vi "SV Limit Test (array) (DBL) (No State).vi"(9 "lower limit":dbl, 10 "upper limit":dbl, 11 "Y":dbl[](array[numeric])) -> (1 "lower":T1, 2 "upper":T2, 3 "test passed":bool)   [LabVIEW 2017]
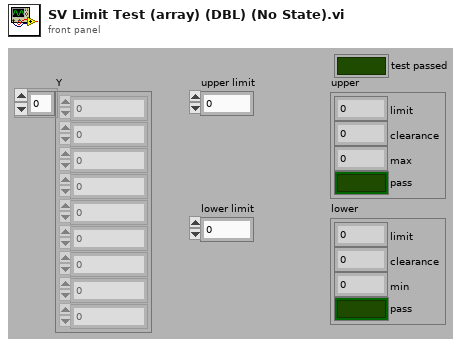
[diagram p1: front panel]
types:
  T1 = cluster{"limit":dbl, "clearance":dbl, "min":dbl, "pass":bool}
  T2 = cluster{"limit":dbl, "clearance":dbl, "max":dbl, "pass":bool}
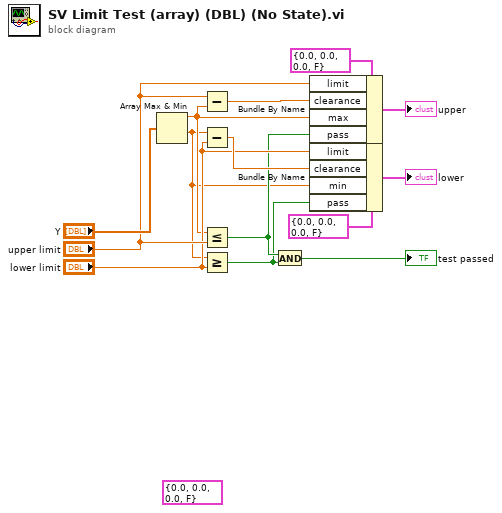
[diagram p0: block diagram]
diagram:
  (unwired) T1 {"limit"=0.0, "clearance"=0.0, "min"=0.0, "pass"=FALSE} ("lower")
  n1 = Array Max & Min(array="Y") -> (max value=w4:dbl, min value=w1:dbl)  [unwired: 2 out]
  n2 = Subtract(x="upper limit", y=w4) -> (x-y=w11:dbl)
  n3 = Subtract(x=w1, y="lower limit") -> (x-y=w7:dbl)
  n4 = Less Or Equal?(x=w4, y="upper limit") -> (x <= y?=w3:bool)
  n5 = Greater Or Equal?(x=w1, y="lower limit") -> (x >= y?=w2:bool)
  n6 = And(x=w3, y=w2) -> (x .and. y?=→"test passed":bool)
  n7 = Bundle By Name(cluster=T2 {"limit"=0.0, "clearance"=0.0, "max"=0.0, "pass"=FALSE} ("upper"), "limit"="upper limit", "clearance"=w11, "max"=w4, "pass"=w3) -> (→"upper":T2)
  n8 = Bundle By Name(cluster=T1 {"limit"=0.0, "clearance"=0.0, "min"=0.0, "pass"=FALSE} ("lower"), "limit"="lower limit", "clearance"=w7, "min"=w1, "pass"=w2) -> (→"lower":T1)
